vi "Symphony 3d_Data_to_2d.vi"(8 "error in (no error)":errorcluster caption="entrée d'erreur (pas d'erreur)", 10 "Image Mode":bool, 11 "RawDataIn":i32[][][](array[numeric])) -> (0 "error out":errorcluster caption="sortie d'erreur", 2 "RawDataOut":i32[][](array[numeric]), 3 "Column":i32, 5 "Row":i32, 7 "Page":i32)   [LabVIEW 2019]
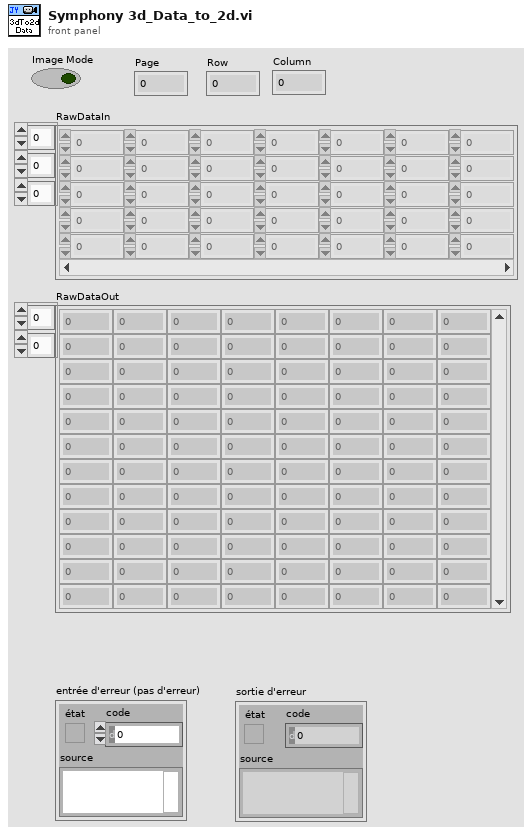
[diagram p1: front panel]
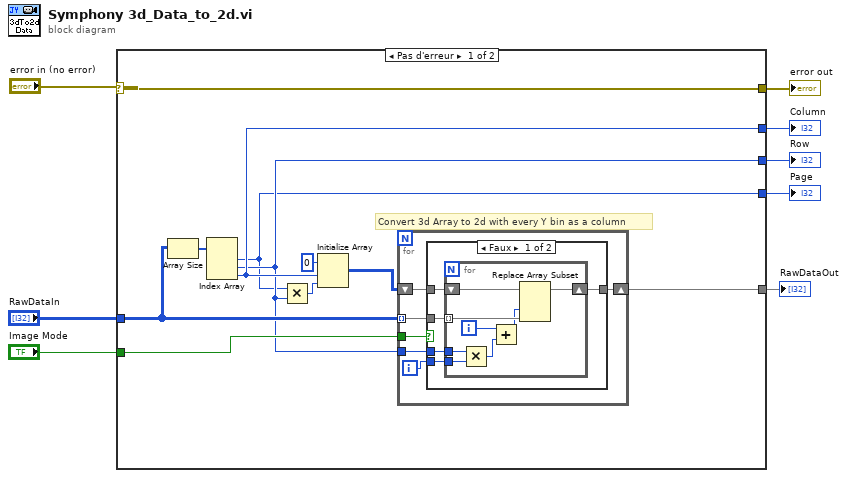
[diagram p0: block diagram]
diagram:
  n1 = case shown="Pas d'erreur" "error in (no error)" {
    selector: "error in (no error)" -> [w13 w40]
    tunnel: "Image Mode" -> [w19 _]
    tunnel: "RawDataIn" -> [w15 _]
    tunnel: [w13 w40] -> w5
    tunnel: [w12 _] -> w4
    tunnel: [w11 _] -> w3
    tunnel: [w10 _] -> w2
    tunnel: [w9 _] -> w1
    frame No Error {
      # "Convert 3d Array to 2d with every Y bin as a column"
      n2 = Array Size(array=w15) -> (size(s)=w18:i32[])
      n3 = Index Array(array=w18) -> (element #1=w10:i32, element #2=w11:i32, element #3=w12:i32)  [unwired: 3 in]
      n4 = Multiply(x=w10, y=w11) -> (x*y=w14:i32)
      n5 = Initialize Array(0 ("élément"), w12, w14) -> (w16:i32[][])
      n6 = for {
        tunnel: w15 -> [w24] mode=indexing
        tunnel: w19 -> [w25]
        shift-right: [w20] -> w9
        shift-left: w16 -> [w23]
        tunnel: w11 -> [w21]
        i -> [w22]
        n7 = case shown="Faux" w25 {
          tunnel: w24 -> [w30 w39]
          tunnel: [w26 w39] -> w20
          tunnel: w23 -> [w29 _]
          tunnel: w22 -> [w28 _]
          tunnel: w21 -> [w27 _]
          frame False {
            n8 = for {
              tunnel: w30 -> [w37] mode=indexing
              tunnel: w28 -> [w36]
              tunnel: w27 -> [w35]
              shift-right: [w32] -> w26
              shift-left: w29 -> [w38]
              i -> [w34]
              n9 = Multiply(x=w35, y=w36) -> (x*y=w33:i32)
              n10 = Add(x=w34, y=w33) -> (x+y=w31:i32)
              n11 = Replace Array Subset(array=w38, new element=w37, index (col)=w31) -> (w32:i32[][])  [unwired: 1 in]
            }
          }
          frame True {
          }
        }
      }
    }
    frame Error {
    }
  }
  "error out" <- w5
  "Page" <- w2
  "Row" <- w3
  "Column" <- w4
  "RawDataOut" <- w1
